vi "LightONjh.vi"() -> ()   [LabVIEW 2015]
uses:
  <vilib>/NXT/Block Support/NXT_InputPort.ctl
  <vilib>/NXT/Block Support/NXT_OutputPort.ctl
  <vilib>/NXT/Dual Mode Library/Sensors/Light_On.vi
  <vilib>/NXT/NXTIO Xnodes/NXTIONodeSubVIs/NXTMoveMotors.vi
  <vilib>/NXT/Dual Mode Library/Waits/Wait_Num.vi
  <vilib>/NXT/Subs/LVHSConnector.ctl
  <vilib>/NXT/NXTIO Xnodes/AddressXNode/NXTIOAddress.xnode
  <vilib>/NXT/NXTIO Xnodes/NXTIOXNode/NXTIO.xnode
  <vilib>/NXT/LegoClasses/BrickReference/BrickReference.lvclass
panel:
  in  "0 speed":i32
  in  "Backward":i32
  in  "Forward":i32
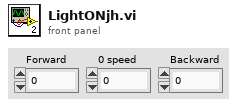
[diagram p1: front panel]
types:
  T1 = typedef "NXT_OutputPort.ctl" = u8
  T2 = typedef "NXT_InputPort.ctl" = u32
  T3 = typedef "LVHSConnector.ctl" = refnum<class "BrickReference.lvclass">
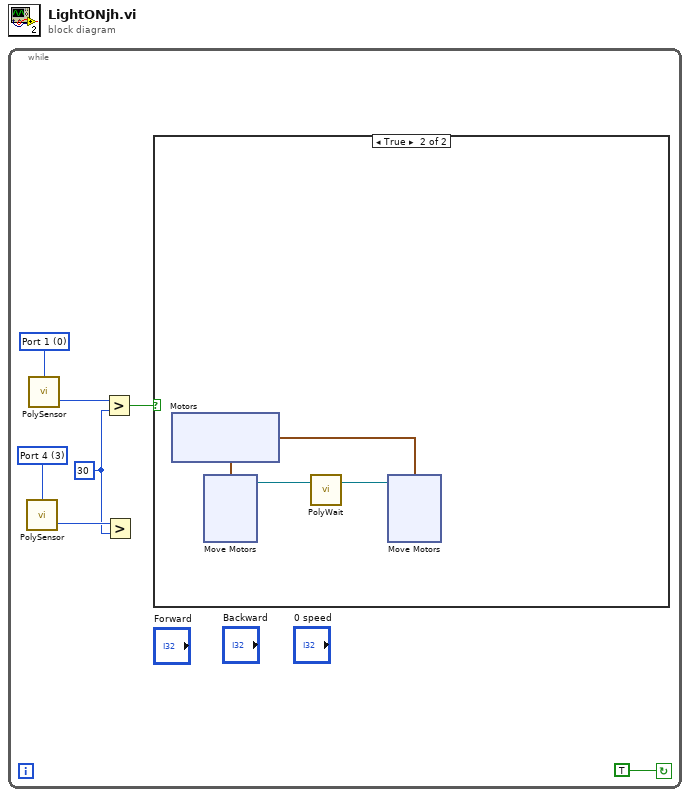
[diagram p0: block diagram]
diagram:
  n1 = while {
    stop <- TRUE continue-if-true
    w3 = 30
    w6 = T2 3 items=["Port 1", "Port 2", "Port 3", "Port 4"] ("Port (Port 3)")
    w7 = T2 0 items=["Port 1", "Port 2", "Port 3", "Port 4"] ("Port (Port 3)")
    n2 = call-poly <vilib>:"PolySensor.vi"("Port (Port 3)"=w6) -> ("Scaled Value"=w5:i16)  [unwired: 2 in, 1 out]
    n3 = call-poly <vilib>:"PolySensor.vi"("Port (Port 3)"=w7) -> ("Scaled Value"=w4:i16)  [unwired: 2 in, 1 out]
    n4 = Greater?(x=w4, y=w3) -> (0:w1:bool)
    n5 = Greater?(x=w5, y=w3) -> ()  [unwired: 1 out]
    n6 = case shown="True" w1 {
      frame False {
      }
      frame True {
        n7 = xnode "Motors"() -> ("Motor"=w10:cluster{"Port":T1, "Port":T1})
        n8 = xnode "Move Motors"("Motors"=w10) -> ("NXT/EV3"=w9:T3)  [unwired: 3 in]
        n9 = call-poly <vilib>:"PolyWait.vi"("NXT/EV3"=w9) -> ("NXT/EV3"=w8:T3)  [unwired: 3 in]
        n10 = xnode "Move Motors"("Motors"=w10, "NXT/EV3"=w8) -> ()  [unwired: 2 in, 1 out]
      }
    }
  }
